vi "simulate-dashboard.vi"() -> ()   [LabVIEW 2019]
uses:
  Swerve_Drive_System/SDO_DRIVE_GLOBALS.vi
  Simulation/SDO_SIM_SIM_Globals.vi
  Trajectory Following/SDO_TRAJECTORY_GLOBALS.vi
  <vilib>/Rock Robotics/WPI/ThirdParty/JAS_Junk/TrajLib/TypeDef/ROTATION2D.ctl
  <vilib>/Rock Robotics/WPI/ThirdParty/JAS_Junk/TrajLib/Trajectory_Library.lvlib
  <vilib>/Rock Robotics/WPI/ThirdParty/JAS_Junk/TrajLib/TypeDef/SWERVE_DRIVE_MODULE_STATE.ctl
  <vilib>/Rock Robotics/WPI/ThirdParty/JAS_Junk/TrajLib/TypeDef/SWERVE_DRIVE_MODULE_POSITION.ctl
  <vilib>/Rock Robotics/WPI/ThirdParty/JAS_Junk/TrajLib/TypeDef/CHASSIS_SPEEDS.ctl
  <vilib>/Rock Robotics/WPI/ThirdParty/JAS_Junk/TrajLib/TypeDef/TRANSLATION2D.ctl
  <vilib>/Rock Robotics/WPI/ThirdParty/JAS_Junk/TrajLib/TypeDef/POSE2D.ctl
  <vilib>/Rock Robotics/WPI/ThirdParty/JAS_Junk/TrajLib/TypeDef/TRAJ_STATE.ctl
panel:
  in  "Tab Control":T1(tab)
  out "Mod Swerve in Deadband 2":bool
  out "Battery Voltage":dbl(graph)
  out "Swerve Motor Demands":T2(graph)
  out "Drive Motor Demands":T2(graph)
  out "Swerve Module Devices":T3(array[cluster])
  out "GyroReading_Degreees":dbl format="%15.3f"
  out "Encoder Distances":dbl[](array[numeric]) format="%17.2f"
  out "Encoder Velocities":dbl[](array[numeric]) format="%17.2f"
  out "Motor Demands":dbl[](array[numeric]) format="%17.2f"
  out "Battery Volts":dbl format="%16.2f"
  out "Swerve Module Positions":T4[](array[typedef]) {"Angle"."SIN" format="%13.4f"; "Angle"."COS" format="%13.4f"; "Angle"."VALUE" format="%13.4f"; "Distance" format="%19.2f"}
  out "Swerve Module States":T6[](array[typedef]) {"Angle"."SIN" format="%13.4f"; "Angle"."COS" format="%13.4f"; "Angle"."VALUE" format="%13.4f"; "Speed" format="%18.2f"}
  out "Adjusted Module State Demands":T6[](array[typedef]) {"Angle"."SIN" format="%13.4f"; "Angle"."COS" format="%13.4f"; "Angle"."VALUE" format="%13.4f"; "Speed" format="%20.2f"}
  out "Orientation Angle Dmd_Rad":dbl format="%17.3f"
  out "Drv Chassis Velocity DmD":T7 {"vOmega" format="%10.3f"; "vY" format="%10.3f"; "vX" format="%10.3f"}
  out "GyroHeading_Radians":dbl format="%17.2f"
  out "Orientation Angle Error_Rad":dbl format="%17.3f"
  out "Orientation Correct CO":dbl format="%17.3f"
  out "Adjusted Chassis Dmd":T7 {"vOmega" format="%10.3f"; "vY" format="%10.3f"; "vX" format="%10.3f"}
  out "Swerve Chassis Speed":T7 {"vOmega" format="%10.3f"; "vY" format="%10.3f"; "vX" format="%10.3f"}
  out "Mod Swerve in Deadband":bool
  out "Trajectory Status":T8(graph)
  out "Trajectory Execution \nClosed Loop":bool
  out "Mod Swerve in \nDeadband 3":bool
  out "Trajectory Error":T9(graph)
  out "Traj_OnTarget":bool
  out "Traj Heading Dmd Deg":dbl format="%17.2f"
  out "Traj Final Heading Dmd Deg":dbl format="%17.2f"
  out "Traj Sample Time Sec":dbl format="%17.2f"
  out "Traj Rot Vel FF Rad/Sec":dbl format="%17.2f"
  out "Relative Trajectory Pose":T10={"TRANSLATION"={"X"=0.0, "Y"=0.0}, "ROTATION"={"VALUE"=0.0, "COS"=1.0, "SIN"=0.0}} {"ROTATION"."SIN" format="%13.4f"; "ROTATION"."COS" format="%13.4f"; "ROTATION"."VALUE" format="%13.4f"; "TRANSLATION"."Y" format="%14.3f"; "TRANSLATION"."X" format="%14.3f"}
  out "Absolute Odometry \nPose":T10={"TRANSLATION"={"X"=0.0, "Y"=0.0}, "ROTATION"={"VALUE"=0.0, "COS"=1.0, "SIN"=0.0}} {"ROTATION"."SIN" format="%13.4f"; "ROTATION"."COS" format="%13.4f"; "ROTATION"."VALUE" format="%13.4f"; "TRANSLATION"."Y" format="%14.3f"; "TRANSLATION"."X" format="%14.3f"}
  out "Current Trajectory State":T12={"TimeSeconds"=0.0, "Velocity"=0.0, "Acceleration"=0.0, "POSE"={"TRANSLATION"={"X"=0.0, "Y"=0.0}, "ROTATION"={"VALUE"=0.0, "COS"=1.0, "SIN"=0.0}}, "Curvature"=0.0} {"POSE"."ROTATION"."SIN" format="%13.4f"; "POSE"."ROTATION"."COS" format="%13.4f"; "POSE"."ROTATION"."VALUE" format="%13.4f"; "POSE"."TRANSLATION"."Y" format="%14.3f"; "POSE"."TRANSLATION"."X" format="%14.3f"}
  out "Other ABS Odometry\nPose":T10={"TRANSLATION"={"X"=0.0, "Y"=0.0}, "ROTATION"={"VALUE"=0.0, "COS"=1.0, "SIN"=0.0}} {"ROTATION"."SIN" format="%13.4f"; "ROTATION"."COS" format="%13.4f"; "ROTATION"."VALUE" format="%13.4f"; "TRANSLATION"."Y" format="%14.3f"; "TRANSLATION"."X" format="%14.3f"}
  # "SIMULATION"
  # "SWERVE DRIVE"
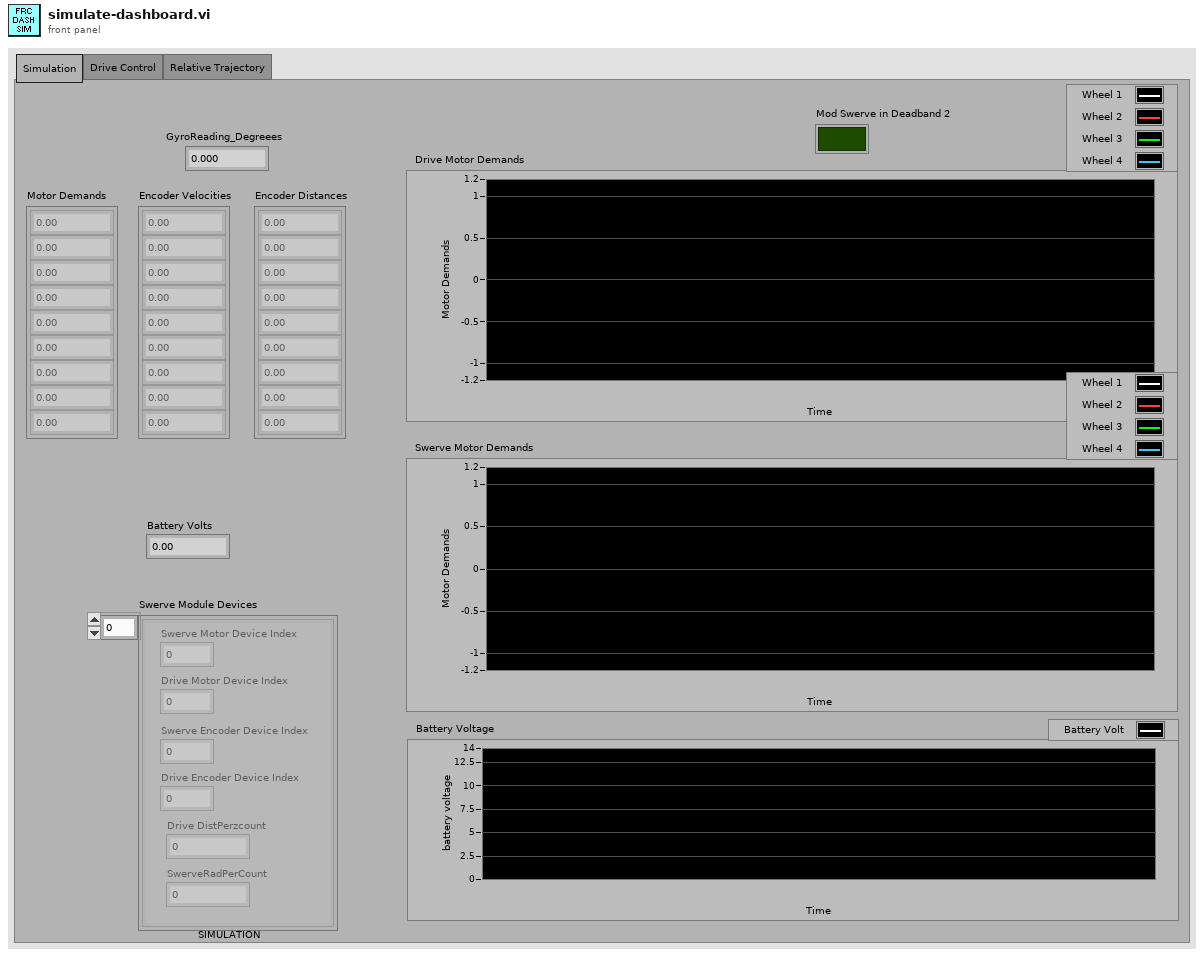
[diagram p1: front panel]
types:
  T1 = enum32{"Simulation", "Drive Control", "Relative Trajectory"}
  T2 = cluster{"Motor Dmd":dbl, "Motor Dmd":dbl, "Motor Dmd":dbl, "Motor Dmd":dbl}
  T3 = cluster{"Swerve Motor Device Index":i32, "Drive Motor Device Index":i32, "Swerve Encoder Device Index":i32, "Drive Encoder Device Index":i32, "Drive DistPerzcount":dbl, "SwerveRadPerCount":dbl}[]
  T4 = typedef "Trajectory_Library.lvlib/SWERVE_DRIVE_MODULE_POSITION.ctl" = cluster{"Distance":dbl, "Angle":T5, "P":bool}
  T5 = typedef "Trajectory_Library.lvlib/ROTATION2D.ctl" = cluster{"VALUE":dbl, "COS":dbl, "SIN":dbl}
  T6 = typedef "Trajectory_Library.lvlib/SWERVE_DRIVE_MODULE_STATE.ctl" = cluster{"Speed":dbl, "Angle":T5}
  T7 = typedef "Trajectory_Library.lvlib/CHASSIS_SPEEDS.ctl" = cluster{"vX":dbl, "vY":dbl, "vOmega":dbl}
  T8 = cluster{dbl, dbl, dbl, "Traj_Sample_Time_Sec":dbl}
  T9 = cluster{"Traj X Err":dbl, "Traj Y Err":dbl, "Traj Heading Err":dbl}
  T10 = typedef "Trajectory_Library.lvlib/POSE2D.ctl" = cluster{"TRANSLATION":T11, "ROTATION":T5}
  T11 = typedef "Trajectory_Library.lvlib/TRANSLATION2D.ctl" = cluster{"X":dbl, "Y":dbl}
  T12 = typedef "Trajectory_Library.lvlib/TRAJ_STATE.ctl" = cluster{"TimeSeconds":dbl, "Velocity":dbl, "Acceleration":dbl, "POSE":T10, "Curvature":dbl}
  T13 = cluster{"Traj X Err_FT":dbl, "Traj Y Err_FT":dbl, "Traj Heading Err_DEG":dbl}
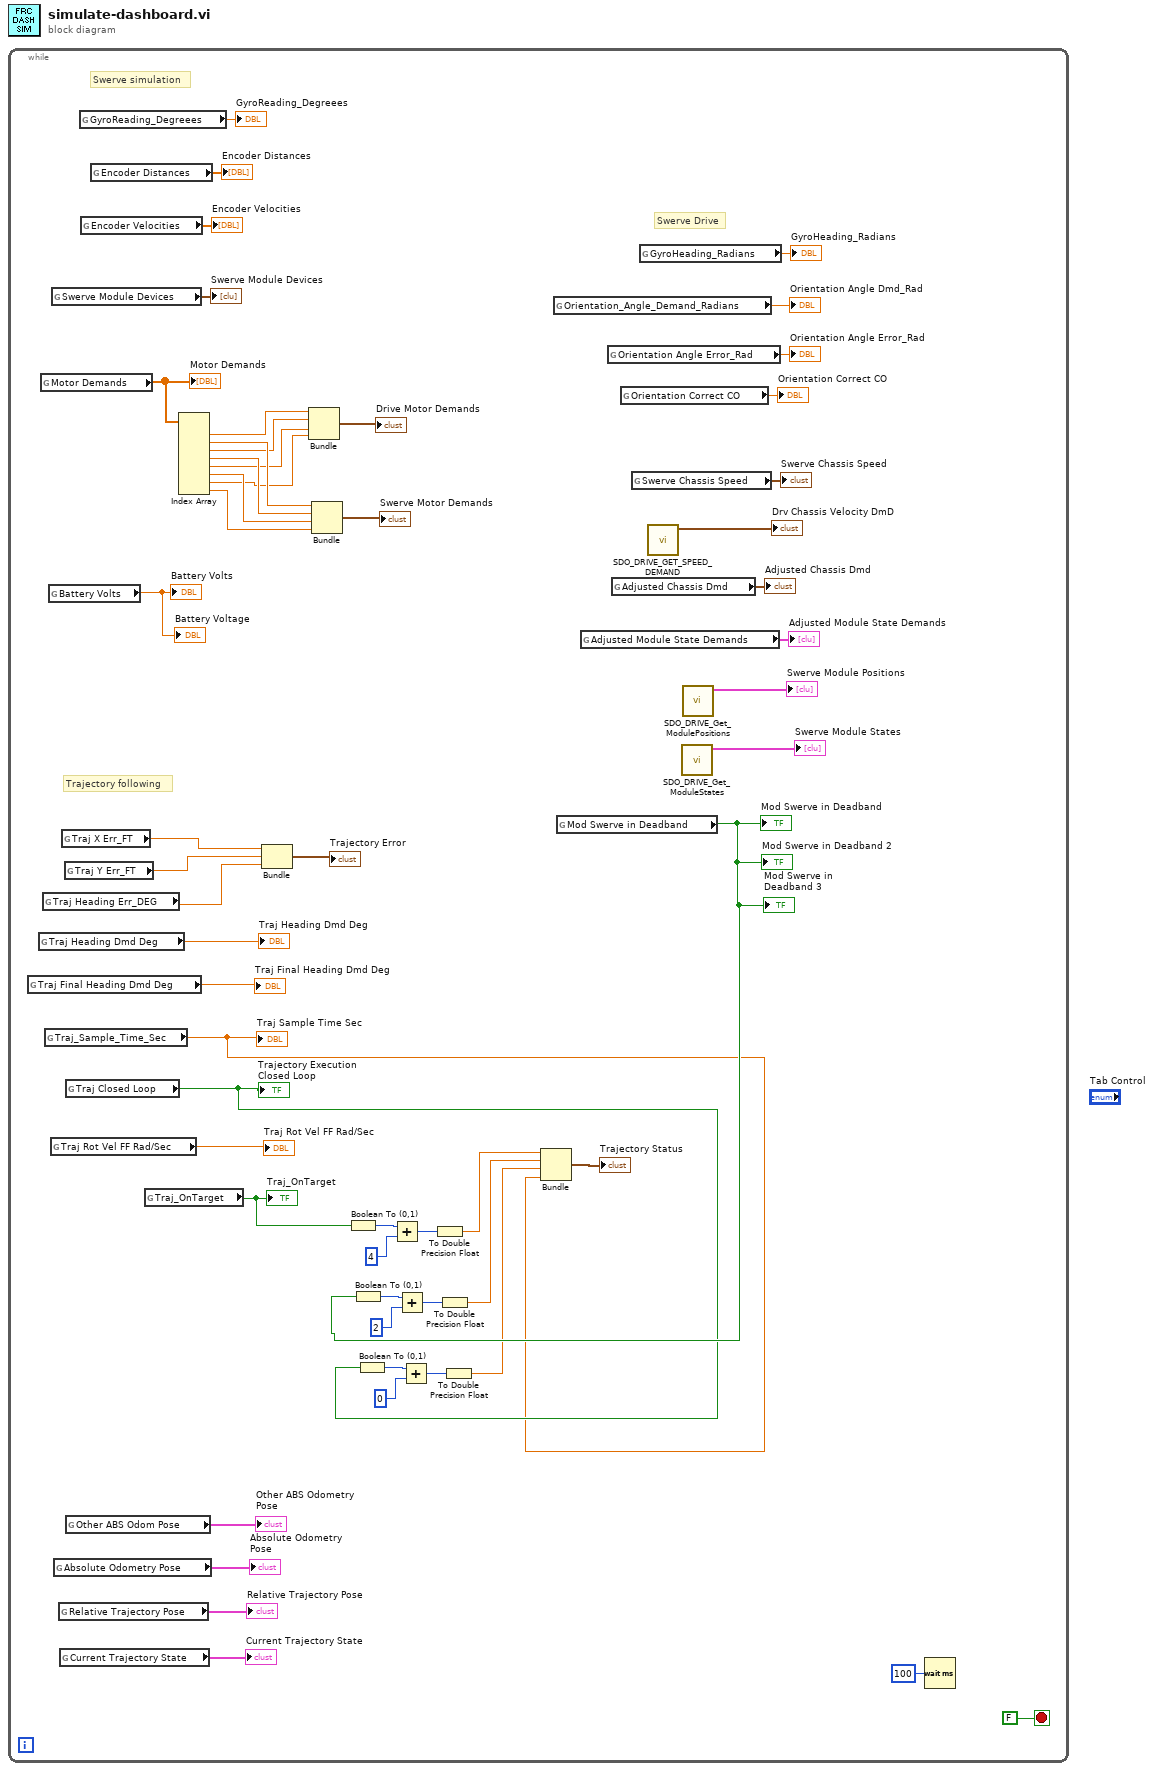
[diagram p0: block diagram]
diagram:
  n1 = while {
    stop <- FALSE stop-if-true
    # "Trajectory following"
    # "Swerve simulation"
    # "Swerve Drive"
    n2 = global read "SDO_TRAJECTORY_GLOBALS.vi" "Traj Final Heading Dmd Deg"() -> (→"Traj Final Heading Dmd Deg":dbl)
    n3 = global read "SDO_TRAJECTORY_GLOBALS.vi" "Traj Heading Dmd Deg"() -> (→"Traj Heading Dmd Deg":dbl)
    n4 = global read "SDO_SIM_SIM_Globals.vi" "Motor Demands"() -> (w39:dbl[])
    "Motor Demands" <- w39
    n5 = global read "SDO_TRAJECTORY_GLOBALS.vi" "Traj Heading Err_DEG"() -> (w26:dbl)
    n6 = global read "SDO_TRAJECTORY_GLOBALS.vi" "Traj_Sample_Time_Sec"() -> (w6:dbl)
    "Traj Sample Time Sec" <- w6
    n7 = global read "SDO_SIM_SIM_Globals.vi" "Battery Volts"() -> (→"Battery Volts" →"Battery Voltage":dbl)
    n8 = global read "SDO_TRAJECTORY_GLOBALS.vi" "Traj Rot Vel FF Rad/Sec"() -> (→"Traj Rot Vel FF Rad/Sec":dbl)
    n9 = global read "SDO_SIM_SIM_Globals.vi" "Swerve Module Devices"() -> (→"Swerve Module Devices":T3)
    n10 = global read "SDO_TRAJECTORY_GLOBALS.vi" "Absolute Odometry Pose"() -> (→"Absolute Odometry \nPose":T10)
    n11 = global read "SDO_TRAJECTORY_GLOBALS.vi" "Relative Trajectory Pose"() -> (→"Relative Trajectory Pose":T10)
    n12 = global read "SDO_TRAJECTORY_GLOBALS.vi" "Current Trajectory State"() -> (→"Current Trajectory State":T12)
    n13 = global read "SDO_TRAJECTORY_GLOBALS.vi" "Traj X Err_FT"() -> (w28:dbl)
    n14 = global read "SDO_TRAJECTORY_GLOBALS.vi" "Traj Y Err_FT"() -> (w27:dbl)
    n15 = global read "SDO_TRAJECTORY_GLOBALS.vi" "Traj Closed Loop"() -> (w8:bool)
    "Trajectory Execution \nClosed Loop" <- w8
    n16 = global read "SDO_TRAJECTORY_GLOBALS.vi" "Other ABS Odom Pose"() -> (→"Other ABS Odometry\nPose":T10)
    n17 = global read "SDO_SIM_SIM_Globals.vi" "GyroReading_Degreees"() -> (→"GyroReading_Degreees":dbl)
    n18 = global read "SDO_SIM_SIM_Globals.vi" "Encoder Velocities"() -> (→"Encoder Velocities":dbl[])
    n19 = global read "SDO_SIM_SIM_Globals.vi" "Encoder Distances"() -> (→"Encoder Distances":dbl[])
    n20 = global read "SDO_TRAJECTORY_GLOBALS.vi" "Traj_OnTarget"() -> (w21:bool)
    "Traj_OnTarget" <- w21
    n21 = Index Array(array=w39) -> (element #1=w38:dbl, element #2=w37:dbl, element #3=w36:dbl, element #4=w35:dbl, element #5=w34:dbl, element #6=w33:dbl, element #7=w32:dbl, element #8=w31:dbl)  [unwired: 8 in]
    n22 = Bundle("Traj X Err_FT"=w28, "Traj Y Err_FT"=w27, "Traj Heading Err_DEG"=w26) -> (→"Trajectory Error":T13)  [unwired: 1 in]
    n23 = Bundle("Motor Dmd"=w38, "Motor Dmd"=w36, "Motor Dmd"=w34, "Motor Dmd"=w32) -> (→"Drive Motor Demands":T2)  [unwired: 1 in]
    n24 = Bundle("Motor Dmd"=w37, "Motor Dmd"=w35, "Motor Dmd"=w33, "Motor Dmd"=w31) -> (→"Swerve Motor Demands":T2)  [unwired: 1 in]
    n25 = Boolean To (0,1)(Boolean=w21) -> (0, 1=w19:i16)
    n26 = Boolean To (0,1)(Boolean=w8) -> (0, 1=w11:i16)
    n27 = Add(x=w19, y=i16 4) -> (x+y=w18:i16)
    n28 = Add(x=w11, y=i16 0) -> (x+y=w10:i16)
    n29 = To Double Precision Float(number=w18) -> (double precision float=w20:dbl)
    n30 = To Double Precision Float(number=w10) -> (double precision float=w7:dbl)
    n31 = global read "SDO_DRIVE_GLOBALS.vi" "Orientation_Angle_Demand_Radians"() -> (→"Orientation Angle Dmd_Rad":dbl)
    n32 = global read "SDO_DRIVE_GLOBALS.vi" "Mod Swerve in Deadband"() -> (w13:bool)
    "Mod Swerve in Deadband" <- w13
    "Mod Swerve in Deadband 2" <- w13
    "Mod Swerve in \nDeadband 3" <- w13
    n33 = Boolean To (0,1)(Boolean=w13) -> (0, 1=w16:i16)
    n34 = Add(x=w16, y=i16 2) -> (x+y=w15:i16)
    n35 = To Double Precision Float(number=w15) -> (double precision float=w12:dbl)
    n36 = Bundle(w20, w12, w7, "Traj_Sample_Time_Sec"=w6) -> (→"Trajectory Status":T8)  [unwired: 1 in]
    n37 = global read "SDO_DRIVE_GLOBALS.vi" "Adjusted Module State Demands"() -> (→"Adjusted Module State Demands":T6[])
    n38 = global read "SDO_DRIVE_GLOBALS.vi" "Orientation Angle Error_Rad"() -> (→"Orientation Angle Error_Rad":dbl)
    n39 = global read "SDO_DRIVE_GLOBALS.vi" "Adjusted Chassis Dmd"() -> (→"Adjusted Chassis Dmd":T7)
    n40 = global read "SDO_DRIVE_GLOBALS.vi" "Orientation Correct CO"() -> (→"Orientation Correct CO":dbl)
    n41 = global read "SDO_DRIVE_GLOBALS.vi" "Swerve Chassis Speed"() -> (→"Swerve Chassis Speed":T7)
    n42 = global read "SDO_DRIVE_GLOBALS.vi" "GyroHeading_Radians"() -> (→"GyroHeading_Radians":dbl)
    n43 = call "SDO_DRIVE_GET_SPEED_DEMAND.vi"() -> ("Drv Chassis Velocity DmD"=→"Drv Chassis Velocity DmD":T7)  [unwired: 11 in]
    n44 = call "SDO_DRIVE_Get_ModuleStates.vi"() -> ("Swerve Module States"=→"Swerve Module States":T6[])  [unwired: 11 in]
    n45 = call "SDO_DRIVE_Get_ModulePositions.vi"() -> ("Swerve Module Positions"=→"Swerve Module Positions":T4[])  [unwired: 11 in]
    n46 = Wait (ms)(milliseconds to wait=u32 100) -> ()  [unwired: 1 out]
  }
